vi "1820_ITC_to_DSC.vi"(0 "str":string[](array[string])=["CLMP"], 1 "str var":refnum<k21>[](array[refnum]), 2 "dbl":dbl[](array[numeric])=[0.0, -0.0, 0.0, 0.91, -0.0002, -0.0003, 81.9328, 94.8099], 3 "dbl var":refnum<k21>[](array[refnum])=["ni.var.psp://housesoftheholy/MNK_18T/1820_ITC_Lambda_Temperature", "ni.var.psp://housesoftheholy/MNK_18T/1820_ITC_Pressure", "ni.var.psp://housesoftheholy/MNK_18T/1820_ITC_Needle_Valve", "ni.var.psp://housesoftheholy/MNK_18T/1820_ITC_Lambda_Temperature_R"]) -> ()   [LabVIEW 2016]
panel:
  # "1820 ITC to DSC"
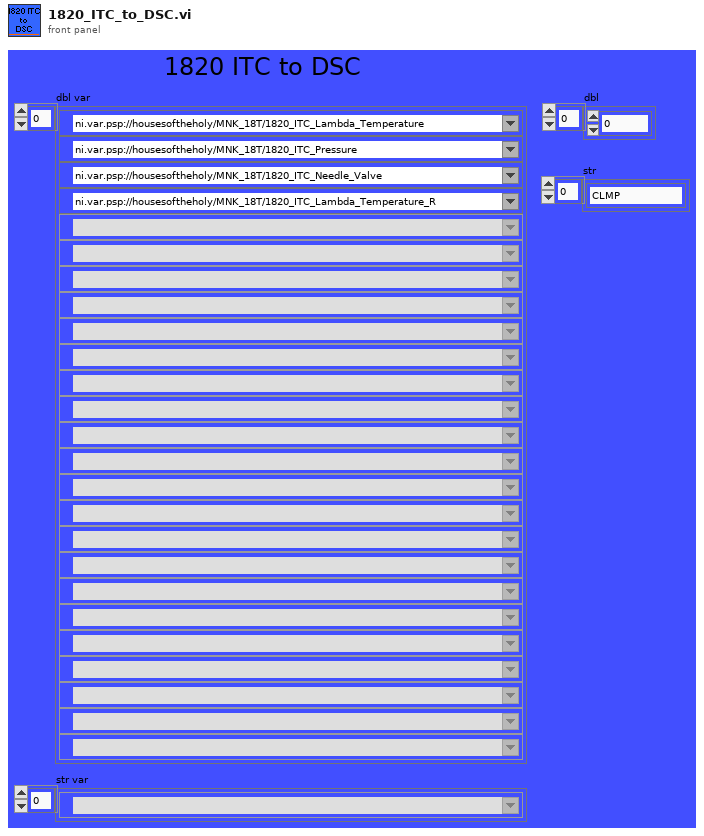
[diagram p1: front panel]
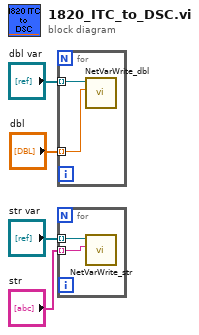
[diagram p0: block diagram]
diagram:
  n1 = for {
    tunnel: "dbl var" -> [w6] mode=indexing
    tunnel: "dbl" -> [w5] mode=indexing
    n2 = call "NetVarWrite_dbl.vi"("Numeric"=w5, "Refnum in"=w6) -> ()  [unwired: 9 in, 1 out]
  }
  n3 = for {
    tunnel: "str var" -> [w8] mode=indexing
    tunnel: "str" -> [w7] mode=indexing
    n4 = call "NetVarWrite_str.vi"("String"=w7, "Refnum in"=w8) -> ()  [unwired: 9 in, 1 out]
  }
